vi "SRNvitezaMCAsimulare.vi"() -> ()   [LabVIEW 2009]
uses:
  <vilib>/ptbypt/NI_PtbyPt.lvlib
panel:
  out "Grafic":cluster{"Valoare de referinta":dbl, dbl}(graph)
  out "Frecventa de esantionare fs(hz)":dbl
  in  "Perioada de esantionare Ts(ms)":dbl
  in  "Perturbatie/Sarcina(RPM)":dbl(slide) scale=-100.0..100.0
  out "Semnal catre element de executie(0 - 10 V)":dbl(slide) scale=0.0..10.0
  out "Display traductor":dbl
  in  "STOP PROCES":bool
  out "PROTECTIE":bool
  out "Avertizare -2%":bool
  out "Avertizare +2%":bool
  out "Vitezometru":dbl(knob) scale=0.0..3000.0
  in  "Valoare de referinta":dbl
  out "Turatie Motor De Curent Alternativ":dbl(knob) scale=0.0..3000.0
  # "PANOU COMANDA"
  # "MONITORIZARE PROCES (MOTOR CA)"
  # "SETARI ACHIZITIE DAQ"
  # "SISTEM DE SIGURANTA"
  # "Timp real"
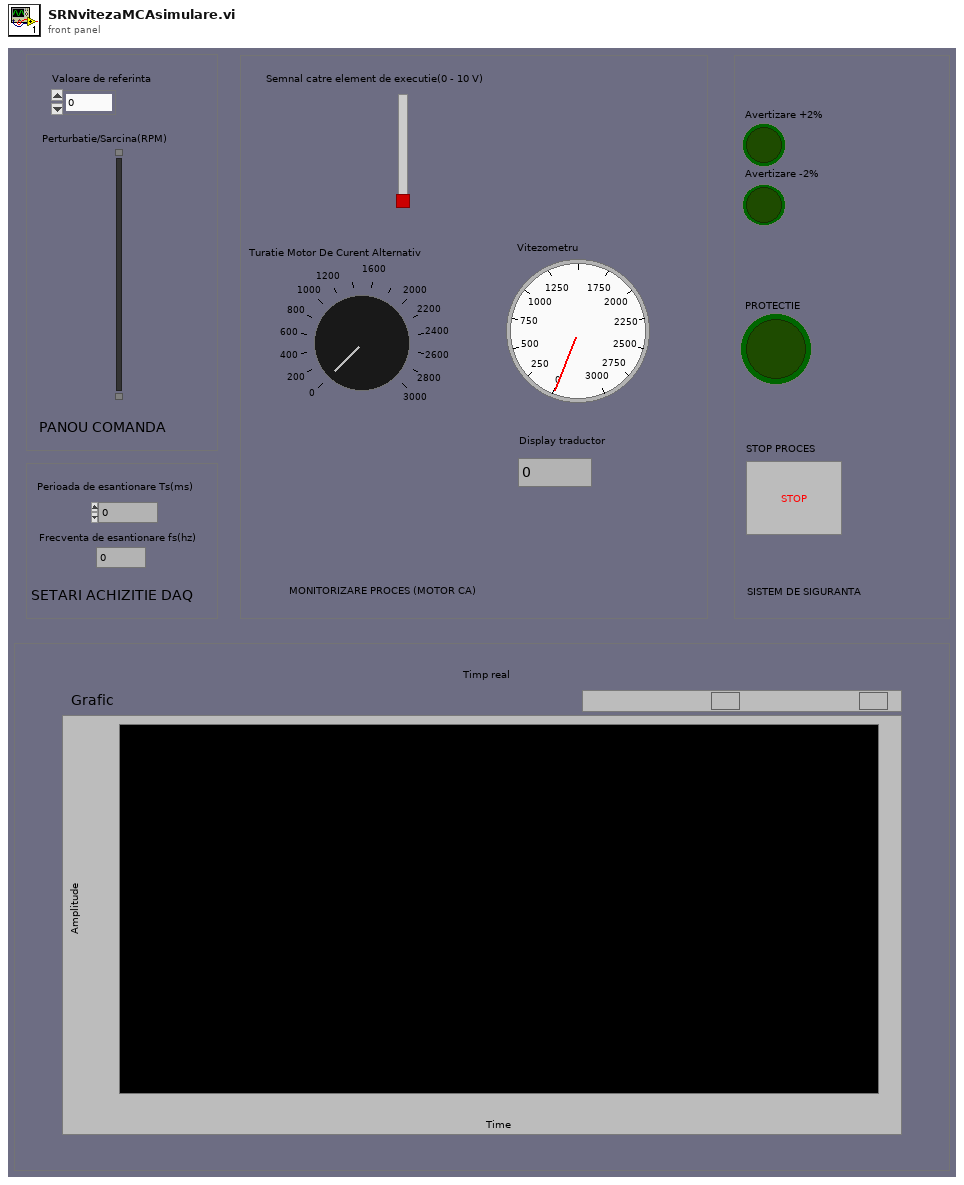
[diagram p1: front panel]
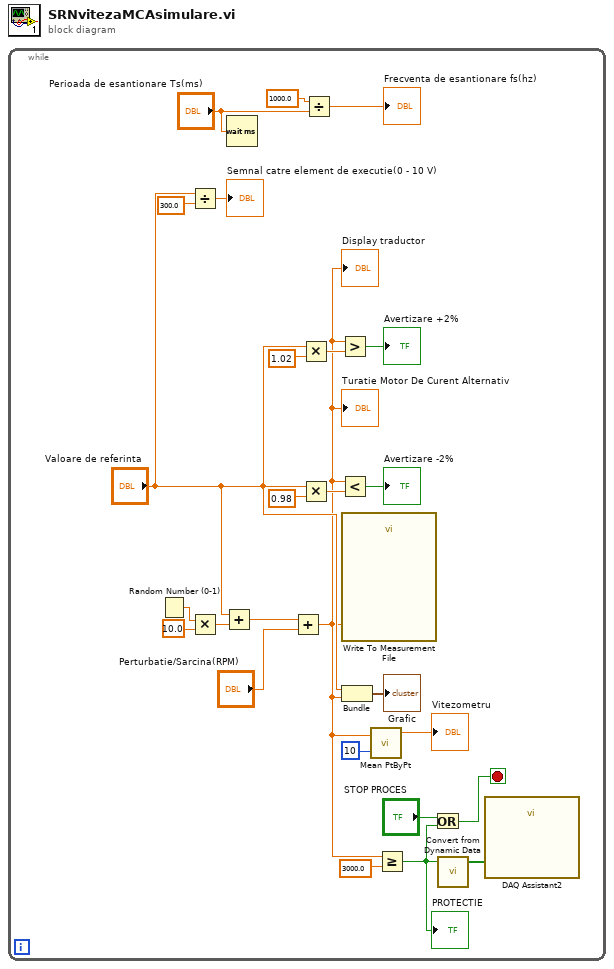
[diagram p0: block diagram]
diagram:
  n1 = while {
    stop <- w18 stop-if-true
    n2 = Random Number (0-1)() -> (number: 0 to 1=w15:dbl)
    n3 = Divide(x="Valoare de referinta", y=300.0 ("x/y")) -> (x/y=→"Semnal catre element de executie(0 - 10 V)":dbl)
    n4 = Multiply(x=w15, y=10.0 ("x")) -> (x*y=w13:dbl)
    n5 = Add(x="Valoare de referinta", y=w13) -> (x+y=w10:dbl)
    n6 = Wait (ms)(milliseconds to wait="Perioada de esantionare Ts(ms)") -> ()  [unwired: 1 out]
    n7 = Add(x=w10, y="Perturbatie/Sarcina(RPM)") -> (x+y=w2:dbl)
    "Turatie Motor De Curent Alternativ" <- w2
    "Display traductor" <- w2
    n8 = Multiply(x="Valoare de referinta", y=1.02) -> (x*y=w24:dbl)
    n9 = Multiply(x="Valoare de referinta", y=0.98) -> (x*y=w22:dbl)
    n10 = Divide(x=1000.0, y="Perioada de esantionare Ts(ms)") -> (x/y=→"Frecventa de esantionare fs(hz)":dbl)
    n11 = Greater?(x=w2, y=w24) -> (0:→"Avertizare +2%":bool)
    n12 = Less?(x=w2, y=w22) -> (x < y?=→"Avertizare -2%":bool)
    n13 = call "Write To Measurement File"("Signals"=w2) -> ()  [unwired: 16 in, 3 out]
    n14 = Bundle("Valoare de referinta"="Valoare de referinta", w2) -> (→"Grafic":cluster{"Valoare de referinta":dbl, dbl})  [unwired: 1 in]
    n15 = call <vilib>:"Mean PtByPt.vi"("x"=w2, "sample length"=10) -> ("mean"=→"Vitezometru":dbl)  [unwired: 2 in, 1 out]
    n16 = Greater Or Equal?(x=w2, y=3000.0) -> (x >= y?=w17:bool)
    "PROTECTIE" <- w17
    n17 = Or(x="STOP PROCES", y=w17) -> (x .or. y?=w18:bool)
    n18 = call "Convert from Dynamic Data"("Dynamic Data Type"=w17) -> ("Array"=w16:bool[])  [unwired: 3 in]
    n19 = call "DAQ Assistant2"("data"=w16) -> ()  [unwired: 17 in, 2 out]
  }
